vi "Test_ParseIDFromAnswer.vi"   [LabVIEW 2023]
uses:
  <vilib>/addons/_JKI Toolkits/Caraya/classes/Test/Test.lvclass
  <vilib>/addons/_JKI Toolkits/Caraya/classes/Assert/Assert.lvclass
  <vilib>/addons/_JKI Toolkits/Caraya/classes/Assert/Assert Equal Value_Variant.vi
  <vilib>/addons/_JKI Toolkits/Caraya/classes/Assert/Assert Not Error.vi
  Classes/Communicator/Communicator.lvclass
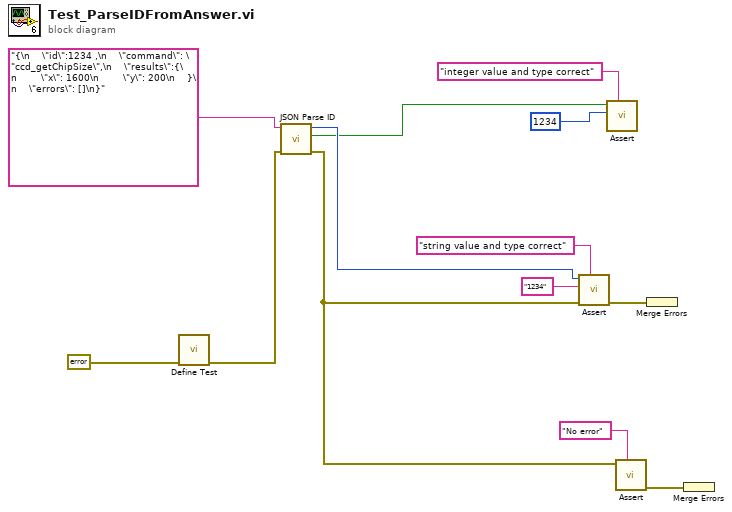
[diagram p0: block diagram]
diagram:
  n1 = call <vilib>:"Define Test.vi"("error in (no error)"=errorcluster {"status"=FALSE, "code"=0, "source"=""}) -> ("error out"=w11:errorcluster)  [unwired: 9 in, 1 out]
  n2 = call "JSON Parse ID.vi"("error in (no error)"=w11, "JSON"="{\n    \"id\":1234 ,\n    \"command\": \"ccd_getChipSize\",\n    \"results\":{\n        \"x\": 1600\n        \"y\": 200\n    }\n    \"errors\": []\n}") -> ("error out"=w10:errorcluster, "key found?"=w1:bool, "ID"=w5:i32)  [unwired: 7 in]
  n3 = call-poly <vilib>:"Assert.vi"("Label"="string value and type correct" ("Label (VI Title)"), "error in (no error)"=w10, "Y"="1234", "X"=w5) -> ("error out"=w8:errorcluster)  [unwired: 6 in, 1 out]
  n4 = call-poly <vilib>:"Assert.vi"("Label"="integer value and type correct" ("Label (VI Title)"), "Y"=1234, "X"=w1) -> ()  [unwired: 7 in, 2 out]
  n5 = call-poly <vilib>:"Assert.vi"("Label"="No error" ("Label (VI Title)"), "Not Error?"=w10) -> ("error out"=w6:errorcluster)  [unwired: 8 in, 1 out]
  n6 = Merge Errors(w8) -> ()  [unwired: 1 out]
  n7 = Merge Errors(w6) -> ()  [unwired: 1 out]
